vi "HXUpdateTerm.vi"(1 "HX State Info":T16 {"BlockNodeState"."Draw Style" items=["FunctionBlock", "ExpressVI", "Variable", "Elemental I/O", "32x32 Icon", "FunctionBlockCompact"]; "BlockNodeState"."Terminal Data"."Terminal Flags" format="%.0b"}, 2 "XNode State Info":T1) -> (0 "BlockNodeState.Terminal Data":T18[](array[typedef]) {"Terminal Flags" format="%.0b"})   [LabVIEW 2017]
uses:
  <vilib>/BlockNodeSupport/TerminalData.ctl
  <vilib>/Platform/storage/lvStorage.llb/xStorage/Write Data/State.ctl
  <vilib>/BlockNodeSupport/BlockNodeState.ctl
  <vilib>/picture/picture.llb/imagedata.ctl
  <vilib>/Platform/storage/lvStorage.llb/dataStorageParams.ctl
  <vilib>/Platform/storage/lvStorage.llb/_selectedProp.ctl
  <vilib>/Platform/storage/lvStorage.llb/dataModel.ctl
  <vilib>/Platform/storage/Storage.llb/usiTypeDef.ctl
  <vilib>/Platform/storage/Storage.llb/usiPropDef.ctl
  <vilib>/express/express shared/ex_EditUserDefinedProperties/usiDataType.ctl
  <vilib>/Platform/storage/Storage.llb/specialProperties.ctl
  <vilib>/Platform/storage/Storage.llb/usiOverwriteOptions.ctl
  <vilib>/Platform/storage/lvStorage.llb/TerminalDef.ctl
  <vilib>/Platform/storage/lvStorage.llb/_TerminalStyle.ctl
  <vilib>/Utility/XNodeSupport.llb/XRect32.ctl
  <vilib>/Platform/storage/Storage.llb/usiSequenceRepresentation.ctl
  <vilib>/Platform/storage/lvStorage.llb/channelType.ctl
  <vilib>/Platform/storage/lvStorage.llb/_dataTerminals.ctl
  <vilib>/Platform/storage/lvStorage.llb/_stateInfoWriteProps.ctl
  <vilib>/Platform/storage/lvStorage.llb/xStorage/Write Data/Write Data.xnode
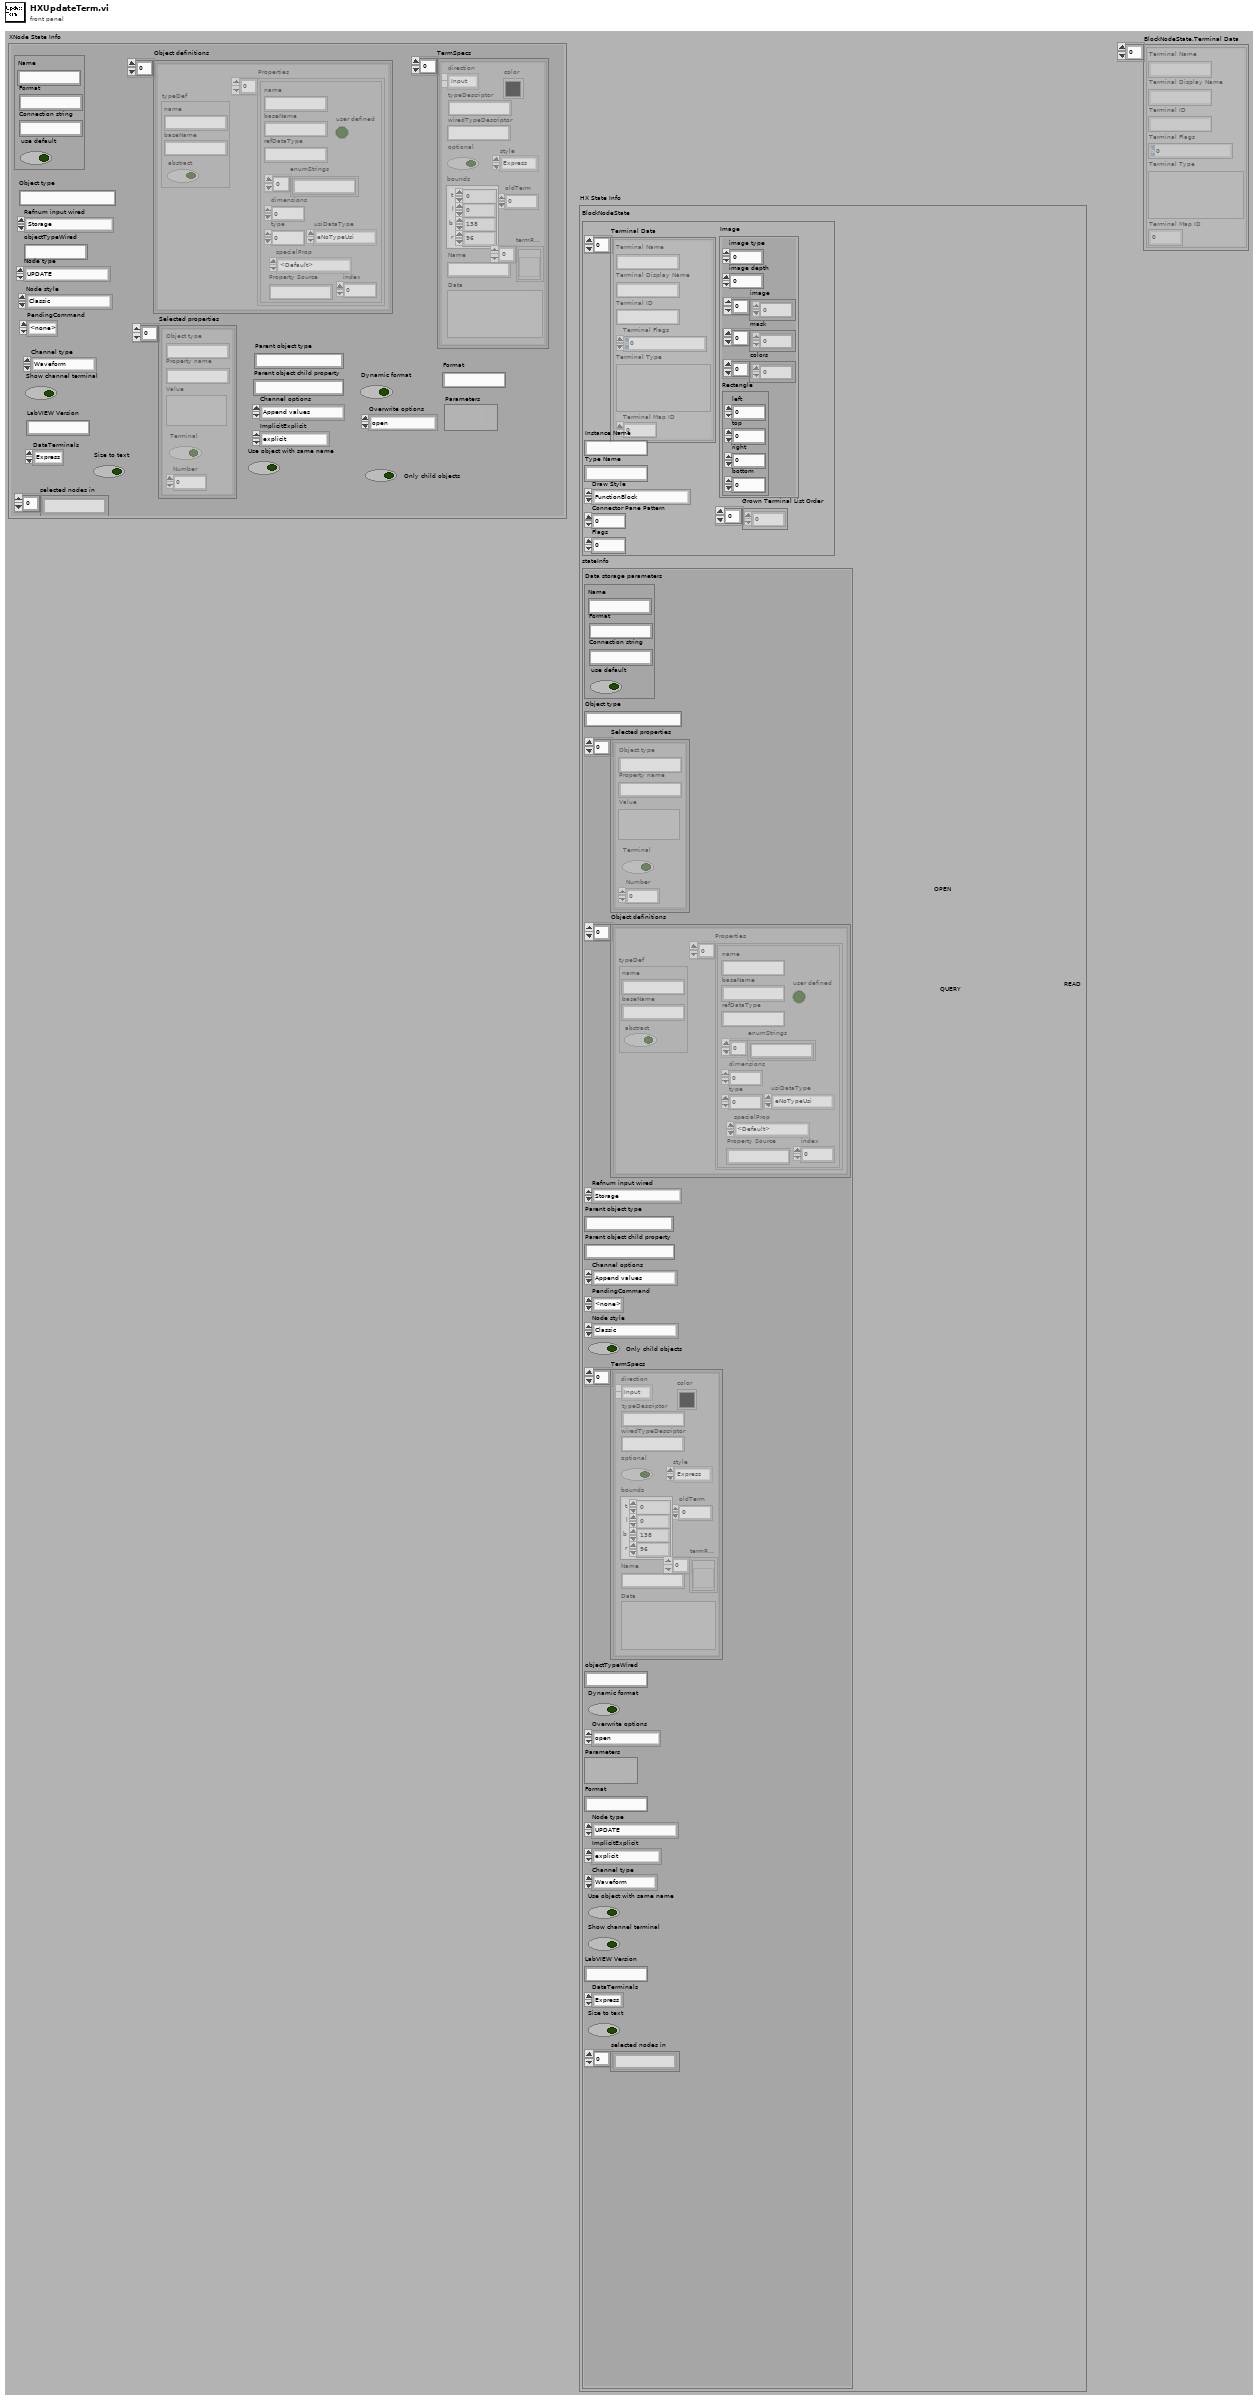
[diagram p1: front panel]
types:
  T1 = typedef "_stateInfoWriteProps.ctl" = cluster{"Data storage parameters":T2, "Object type":string, "Selected properties":T3[], "Object definitions":T4[], "Refnum input wired":enum16{"Storage", "Generic object", "Typed object", "<none>"}, "Parent object type":string, "Parent object child property":string, "Channel options":T9, "PendingCommand":enum16{"<none>", "SelPopUp", "Init"}, "Node style":enum16{"Classic", "Express"}, "Only child objects":bool, "TermSpecs":T10[], "objectTypeWired":string, "Dynamic format":bool, "Overwrite options":enum16{"open", "open or create", "create or replace", "create", "open (read only)"}, "Parameters":variant, "Format":string, "Node type":enum16{"UPDATE", "READ", "QUERY", "CREATE CHILD", "CREATE", "CONNECT", "DISCONNECT"}, "ImplicitExplicit":T13, "Channel type":T14, "Use object with same name":bool, "Show channel terminal":bool, "LabVIEW Version":string, "DataTerminals":T15, "Size to text":bool, "selected nodes in":string[]}
  T2 = typedef "dataStorageParams.ctl" = cluster{"Name":string, "Format":string, "Connection string":string, "use default":bool}
  T3 = typedef "_selectedProp.ctl" = cluster{"Object type":string, "Property name":string, "Value":variant, "Terminal":bool, "Number":i32}
  T4 = typedef "dataModel.ctl" = cluster{"typeDef":T5, "Properties":T6[]}
  T5 = typedef "usiTypeDef.ctl" = cluster{"name":string, "baseName":string, "abstract":bool}
  T6 = typedef "usiPropDef.ctl" = cluster{"name":string, "baseName":string, "refDataType":string, "dimensions":i32, "type":i32, "user defined":bool, "enumStrings":string[], "usiDataType":T7, "specialProp":T8, "Property Source":string, "index":i32}
  T7 = typedef "usiDataType.ctl" = enum16{"eNoTypeUsi", "eInt8Usi", "eInt16Usi", "eInt32Usi", "eInt64Usi", "eUInt8Usi", "eUInt16Usi", "eUInt32Usi", "eUInt64Usi", "eFloat32Usi", "eFloat64Usi", "- 0", "- 1", "- 2", "- 3", "- 4", "- 5", "- 6", "- 7", "- 8", "- 9", "eString8Usi", "eString16Usi", "eStringUsi", "eEnumUsi", "- 10", "- 11", "- 12", "- 13", "- 14", "eTimeUsi", "- 15", "- 16", "- 17", "- 18", "- 19", "- 20", "- 21", "- 22", "- 23", "eInstanceUsi", "eStoreUsi"}
  T8 = typedef "specialProperties.ctl" = enum16{"<Default>", "Channel Values", "AppendReplace", "ChannelFlags", "ValueFlags", "ImplicitExplicit", "InsertIndex", "ValuesCount", "ComparisonOperator", "Cluster", "DAQmx Channel"}
  T9 = typedef "usiOverwriteOptions.ctl" = enum16{"Append values", "Replace values at index", "Replace all values", "Append if timeline aligns"}
  T10 = typedef "TerminalDef.ctl" = cluster{"direction":enum16{"Input", "Output"}, "typeDescriptor":string, "color":u32, "oldTerm":i32, "style":T11, "optional":bool, "bounds":T12, "termRefs":refnum<vi>[], "Name":string, "Data":variant, "wiredTypeDescriptor":string}
  T11 = typedef "_TerminalStyle.ctl" = enum16{"Express", "Collapsed", "Internal"}
  T12 = typedef "XRect32.ctl" = cluster{"t":i32, "l":i32, "b":i32, "r":i32}
  T13 = typedef "usiSequenceRepresentation.ctl" = enum16{"explicit", "implicit"}
  T14 = typedef "channelType.ctl" = enum16{"Waveform", "Array of Double", "Array of String", "DDT", "Array of UInt8", "Array of Int16", "Array of Int32", "Array of Single", "Array of DateTime", "Array of Waveform", "none", "DateTime", "String", "Double", "Single", "UInt8", "Int16", "Int32"}
  T15 = typedef "_dataTerminals.ctl" = enum16{"Express", "Cluster"}
  T16 = typedef "Write Data.xnode/State.ctl" = cluster{"BlockNodeState":T17, "stateInfo":cluster{"Data storage parameters":T2, "Object type":string, "Selected properties":T3[], "Object definitions":T4[], "Refnum input wired":enum16{"Storage", "Generic object", "Typed object", "<none>"}, "Parent object type":string, "Parent object child property":string, "Channel options":T9, "PendingCommand":enum16{"<none>", "SelPopUp", "Init"}, "Node style":enum16{"Classic", "Express"}, "Only child objects":bool, "TermSpecs":T10[], "objectTypeWired":string, "Dynamic format":bool, "Overwrite options":enum16{"open", "open or create", "create or replace", "create", "open (read only)"}, "Parameters":variant, "Format":string, "Node type":enum16{"UPDATE", "READ", "QUERY", "CREATE CHILD", "CREATE", "CONNECT", "DISCONNECT"}, "ImplicitExplicit":T13, "Channel type":T14, "Use object with same name":bool, "Show channel terminal":bool, "LabVIEW Version":string, "DataTerminals":T15, "Size to text":bool, "selected nodes in":string[]}}
  T17 = typedef "BlockNodeState.ctl" = cluster{"Terminal Data":T18[], "Instance Name":string, "Type Name":string, "Draw Style":i32, "Connector Pane Pattern":i32, "Flags":i32, "Grown Terminal List Order":i32[], "Image":T19}
  T18 = typedef "TerminalData.ctl" = cluster{"Terminal Name":string, "Terminal Display Name":string, "Terminal ID":string, "Terminal Flags":i32, "Terminal Type":variant, "Terminal Map ID":i32}
  T19 = typedef "imagedata.ctl" = cluster{"image type":i32, "image depth":i32, "image":u8[], "mask":u8[], "colors":u32[], "Rectangle":cluster{"left":i16, "top":i16, "right":i16, "bottom":i16}}
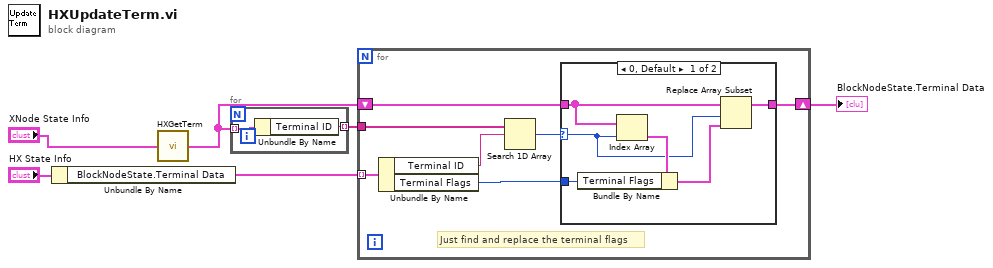
[diagram p0: block diagram]
diagram:
  n1 = Unbundle By Name("HX State Info") -> ("BlockNodeState.Terminal Data"=w5:T18[])
  n2 = call <vilib>:"HXGetTerm.vi"("stateInfoUSIConnect out"="XNode State Info") -> ("BlockNodeState.Terminal Data"=w3:T18[])
  n3 = for {
    tunnel: w3 -> [w8] mode=indexing
    tunnel: [w7] -> w4 mode=indexing
    n4 = Unbundle By Name(w8) -> ("Terminal ID"=w7:string)
  }
  n5 = for {
    tunnel: w5 -> [w15] mode=indexing
    tunnel: w4 -> [w14]
    shift-right: [w10] -> w2
    shift-left: w3 -> [w12]
    # "Just find and replace the terminal flags"
    n6 = Unbundle By Name(w15) -> ("Terminal ID"=w9:string, "Terminal Flags"=w11:i32)
    n7 = Search 1D Array(1D array=w14, element=w9) -> (index of element=w13:i32)  [unwired: 1 in]
    n8 = case shown="0, Default" w13 {
      selector: w13 -> [w18 _]
      tunnel: w12 -> [w19 w22]
      tunnel: [w16 w22] -> w10
      tunnel: w11 -> [w20 _]
      frame 0, Default {
        n9 = Index Array(array=w19, index=w18) -> (element=w21:T18)
        n10 = Bundle By Name(cluster=w21, "Terminal Flags"=w20) -> (w17:T18)
        n11 = Replace Array Subset(array=w19, new element=w17, index=w18) -> (w16:T18[])
      }
      frame -1 {
      }
    }
  }
  "BlockNodeState.Terminal Data" <- w2
